vi "Drive to Image Height (Autonomous).vi"(1 "Execute":bool=TRUE, 2 "Image Height (Pixels)":dbl=10.0, 3 "Percent Velocity":dbl=0.8, 5 "Extra Correction":dbl, 6 "Camera Stabilized?":bool) -> (4 "Done Executing":bool)   [LabVIEW 2011]
uses:
  Globals/Autonomous Joystick Emulation.vi
  Globals/Image Height.vi
  Globals/Alignment Error.vi
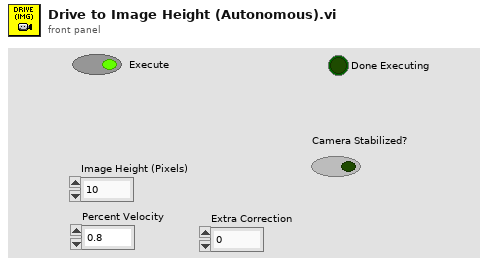
[diagram p1: front panel]
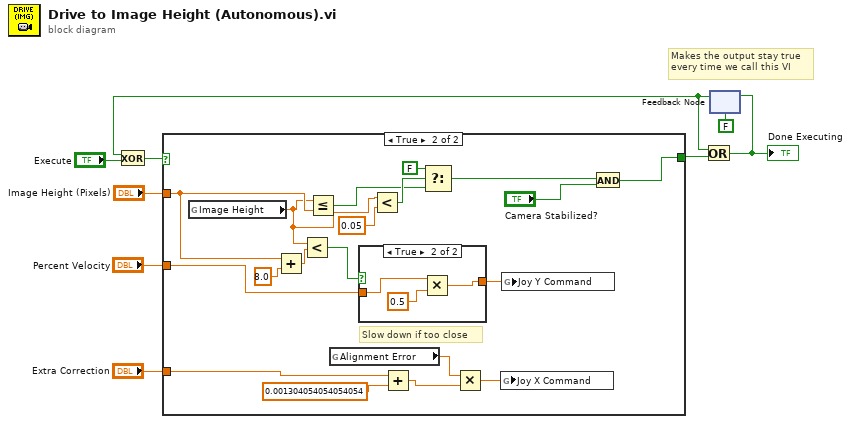
[diagram p0: block diagram]
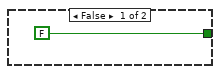
[diagram p2: hidden frame]
diagram:
  # "Makes the output stay true\nevery time we call this VI"
  n1 = feedback #1(FALSE) -> (w4:bool)
  n2 = Exclusive Or(1:"Execute", 2:w4) -> (0:w9:bool)
  n3 = case shown="True" w9 {
    tunnel: [FALSE w14] -> w7
    tunnel: "Percent Velocity" -> [_ w27]
    tunnel: "Image Height (Pixels)" -> [_ w21]
    tunnel: "Extra Correction" -> [_ w11]
    frame False {
    }
    frame True {
      # "Slow down if too close"
      n4 = global read "Image Height.vi" "Image Height"() -> (w16:dbl)
      n5 = Add(x=w21, y=8.0) -> (x+y=w25:dbl)
      n6 = Less?(x=w16, y=w25) -> (x < y?=w29:bool)
      n7 = Less Or Equal?(x=w16, y=w21) -> (x <= y?=w18:bool)
      n8 = global read "Alignment Error.vi" "Alignment Error"() -> (w23:dbl)
      n9 = case shown="True" w29 {
        tunnel: [w30 w31] -> w28
        tunnel: w27 -> [w30 w33]
        frame False {
        }
        frame True {
          n10 = Multiply(x=w33, y=0.5) -> (x*y=w31:dbl)
        }
      }
      n11 = Less?(x=w16, y=0.05) -> (x < y?=w19:bool)
      n12 = Add(x=w11, y=0.001304054054054054 ("Proportional Gain (Alignment)")) -> (x+y=w12:dbl)
      n13 = Select(t=FALSE, s=w19, f=w18) -> (s? t:f=w15:bool)
      n14 = Multiply(x=w23, y=w12) -> (x*y=w22:dbl)
      n15 = global write "Autonomous Joystick Emulation.vi" "Joy X Command"(w22) -> ()
      n16 = global write "Autonomous Joystick Emulation.vi" "Joy Y Command"(w28) -> ()
      n17 = And(x=w15, y="Camera Stabilized?") -> (x .and. y?=w14:bool)
    }
  }
  n18 = Or(x=w4, y=w7) -> (x .or. y?=w3:bool)
  "Done Executing" <- w3
  n19 = feedback-in #1(w3) -> ()
